vi "Method FQN TO Tree Tag.vi"(2 "Message Type":T1, 3 "Method FQN":string) -> (1 "Method Tree Tag":string)   [LabVIEW 2023, in "Message Maker.lvclass"]
uses:
  Message Maker.lvclass
  Message Maker.lvclass/Message Maker.ctl
  Message Type.ctl
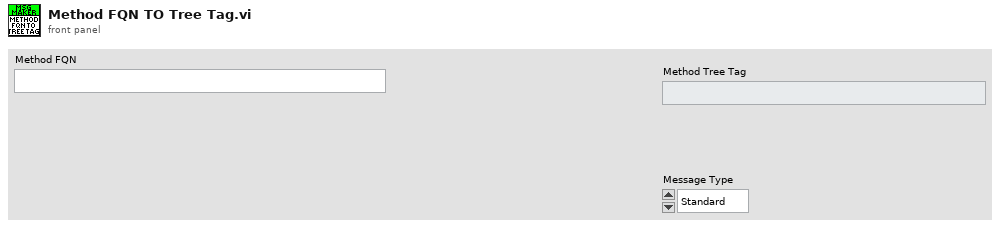
[diagram p1: front panel]
types:
  T1 = typedef "Message Maker.lvclass/Message Type.ctl" = enum16{"Standard", "Async"}
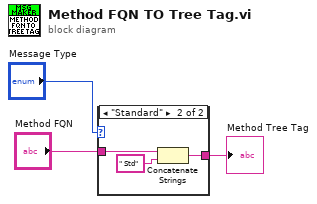
[diagram p0: block diagram]
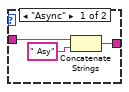
[diagram p2: hidden frame]
diagram:
  n1 = case shown="\"Standard\"" "Message Type" {
    tunnel: "Method FQN" -> [w6 w9]
    tunnel: [w4 w7] -> w1
    frame "Async" {
      n2 = Concatenate Strings(w6, " Asy" ("string")) -> (w4:string)
    }
    frame "Standard" {
      n3 = Concatenate Strings(w9, " Std" ("string")) -> (w7:string)
    }
  }
  "Method Tree Tag" <- w1
